vi "Programing Falsh.vi"() -> ()   [LabVIEW 2018]
uses:
  Typedefs/Command.ctl
  Sub'VIs/Typedefs/CaseControl.ctl
  <vilib>/xnet/xnet.llb/XNET Frame CAN.ctl
  <vilib>/xnet/xnet.llb/XNET Frame Type CAN.ctl
panel:
  in  "exit":bool
  out "Ops":string
  in  "CAN Interface":refnum<k21>="CAN1"
  in  "Start":bool
  in  "path":path
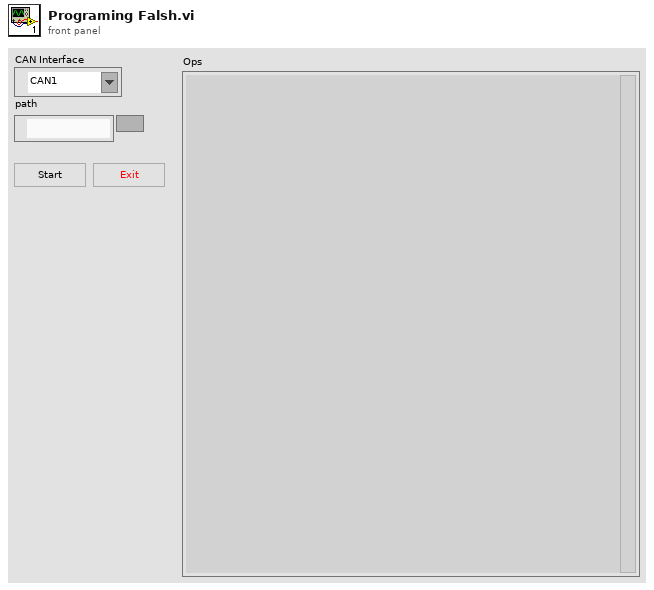
[diagram p1: front panel]
types:
  T1 = typedef "Command.ctl" = enum16{"Extend Session: 10 83", "Tester Present: 3E 80", "Resquest Seed: 27 01", "Send Key: 27 02", "Check FBL:  31 01 FD 02", "Control DTC: 85 82", "Comm Control: 28 83 01", "Program Session Request: 10 02", "Request Seed: 27 35", "Seed Key: 27 36", "Request Download: 34 00 44", "Transfer Data: 36 XX YY", "More Data?", "Request Transfer Exit: 37", "Check Flash Driver Validity: 01 FD 03", "More Segment?", "Write Data Fingereint: 23 F1 F0+26", "EraseFlashMemory Routine: 31 01 FD 00 44", "More segment?(each file)", "CheckAppSwAppData Validity: 31 01 FD 04 44", "CheckAppSwAppData Dependency: 31 01 fd 01", "ECU Reset: 11 81", "System: Init", "System: Idle", "System: Error", "System: Wait", "System: Delay", "System: CAN Send", "System: Exit"}
  T2 = typedef "CaseControl.ctl" = cluster{"histCase":cluster{"time":string, "event":T1, "pass?":bool}[], "retryCount":i32, "lastCase":T1, "nextEvent":T1}
  T3 = cluster{"Write Session in":refnum<k21>, "Read Session in":refnum<k21>, "TxRx Data":string[][], "Response Good?":bool, "spreadsheet string":string, "Rx Message":u8[]}
  T4 = cluster{"path":path, "CAN":cluster{"Write Session in":refnum<k21>, "Read Session in":refnum<k21>, "TxRx Data":string[][], "Response Good?":bool, "spreadsheet string":string, "Rx Message":u8[]}, "error":errorcluster, "CaseControl":T2, "Delay_ms":i32, "Nextevent":T1}
  T5 = typedef "XNET Frame CAN.ctl" = cluster{"timestamp":timestamp, "payload":u8[], "identifier":u32, "type":T6, "extended?":bool, "echo?":bool}
  T6 = typedef "XNET Frame Type CAN.ctl" = u8
  T7 = cluster{"time":string, "event":T1, "pass?":bool}[]
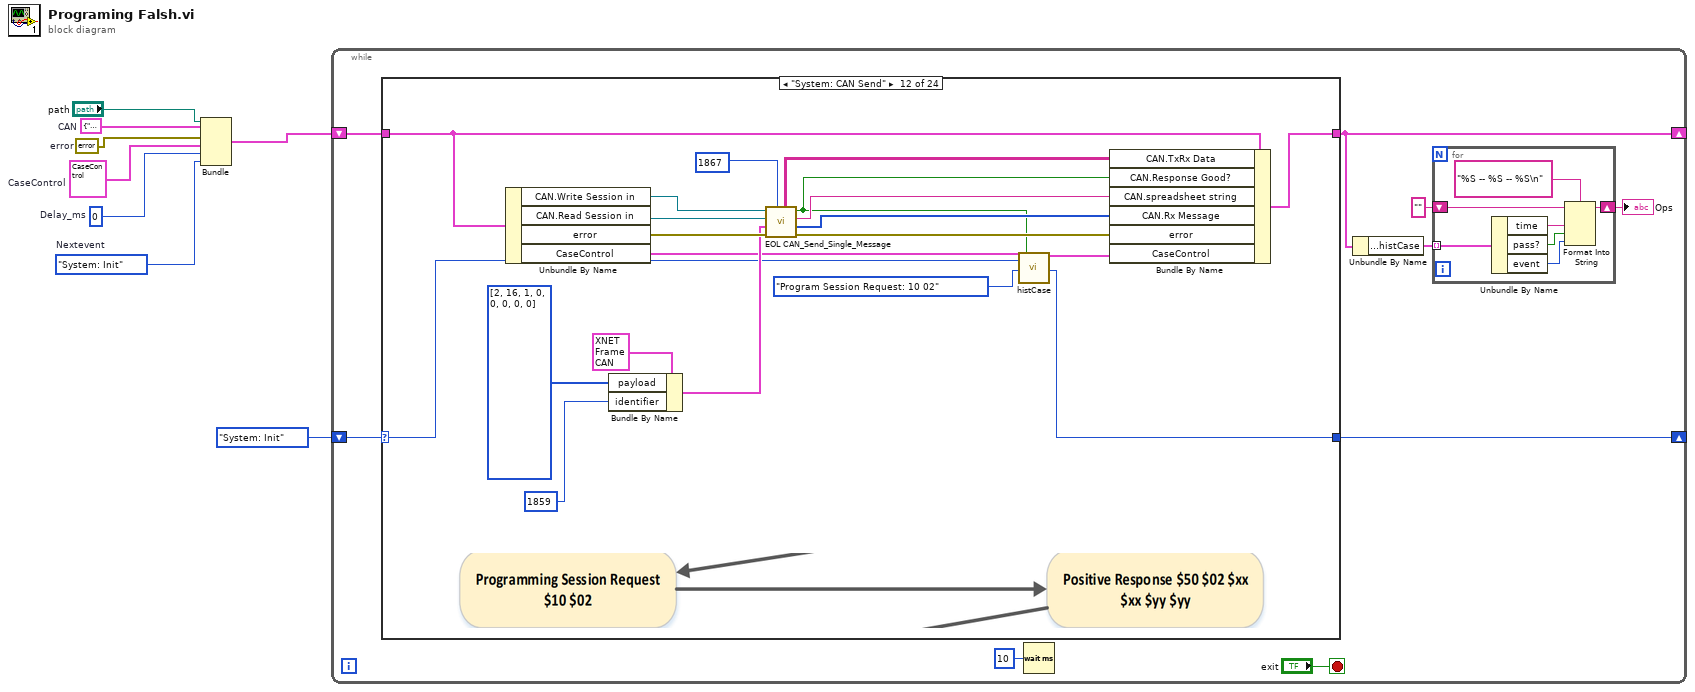
[diagram p0: block diagram]
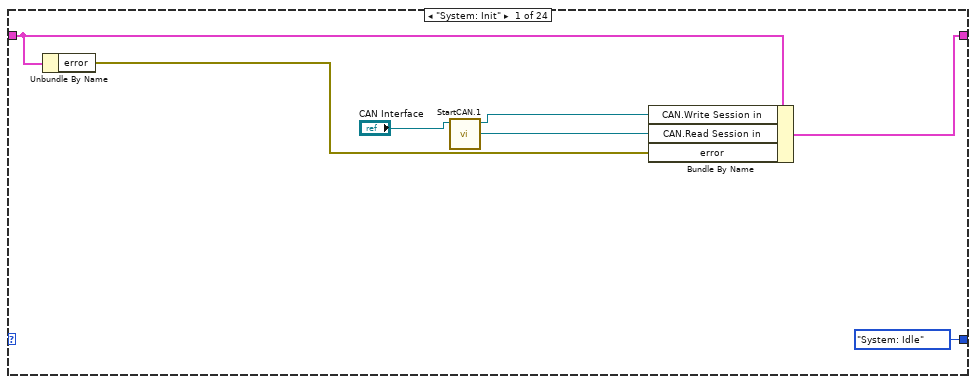
[diagram p2: hidden frame]
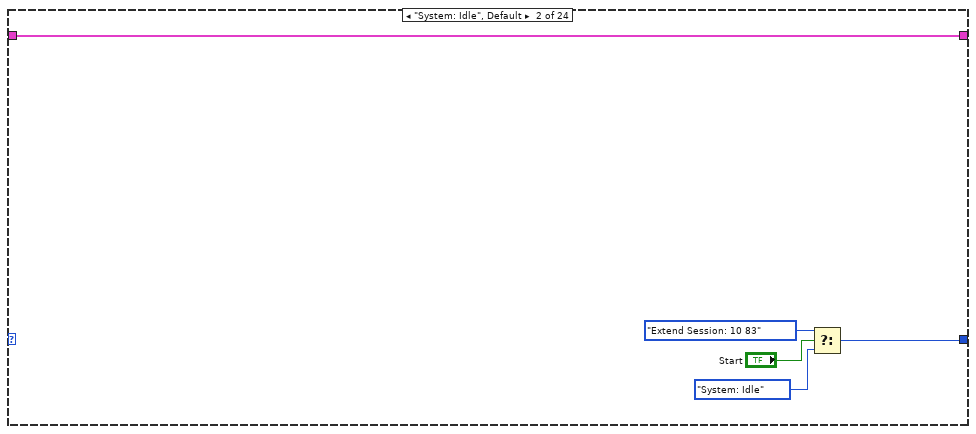
[diagram p3: hidden frame]
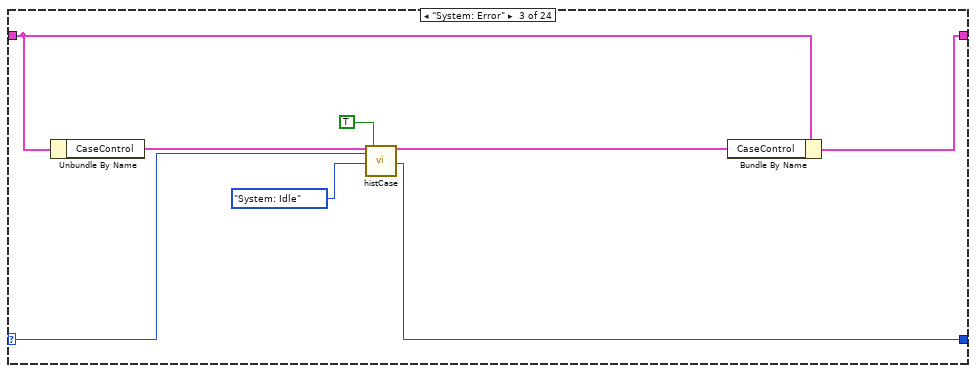
[diagram p4: hidden frame]
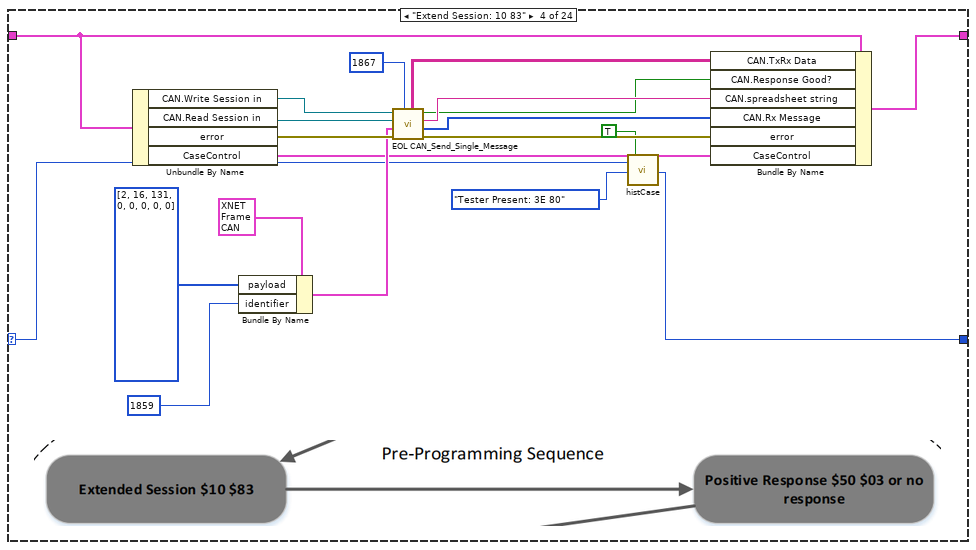
[diagram p5: hidden frame]
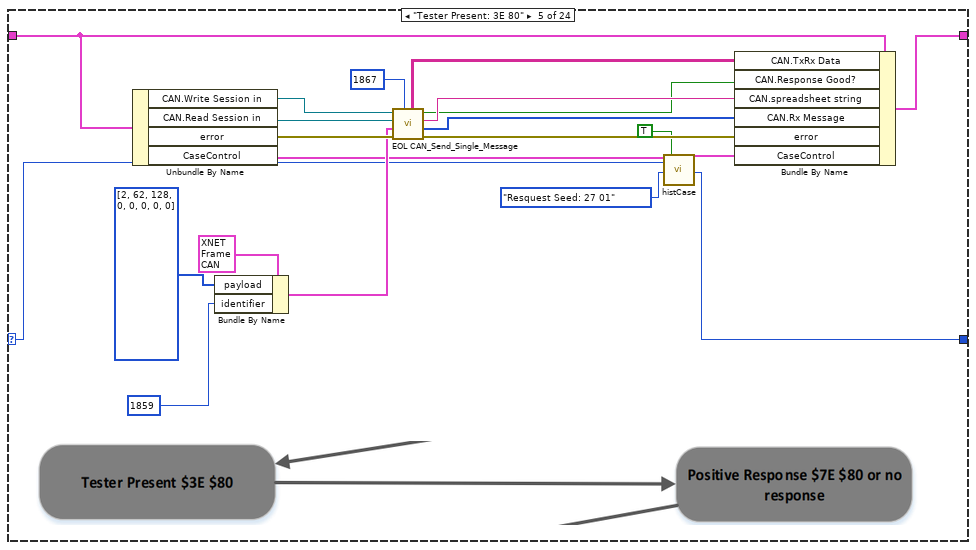
[diagram p6: hidden frame]
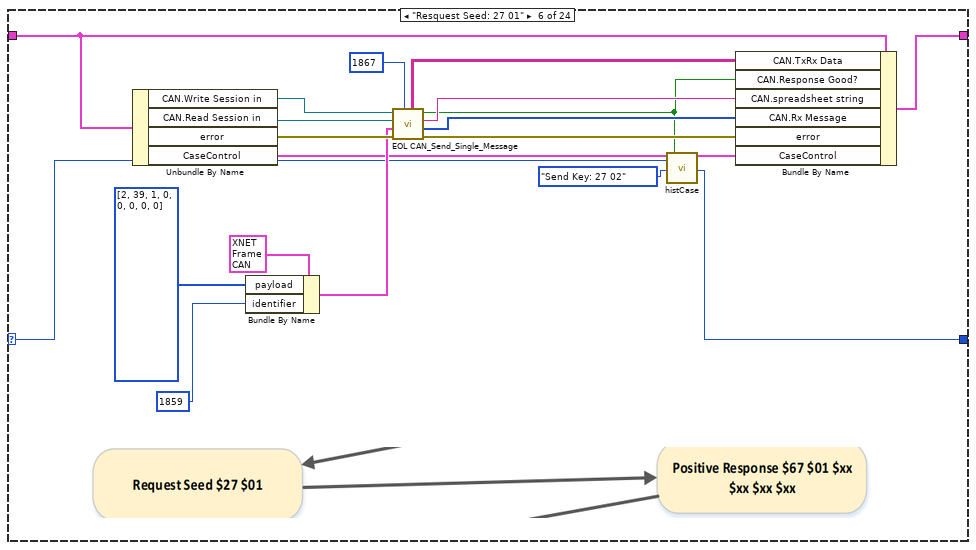
[diagram p7: hidden frame]
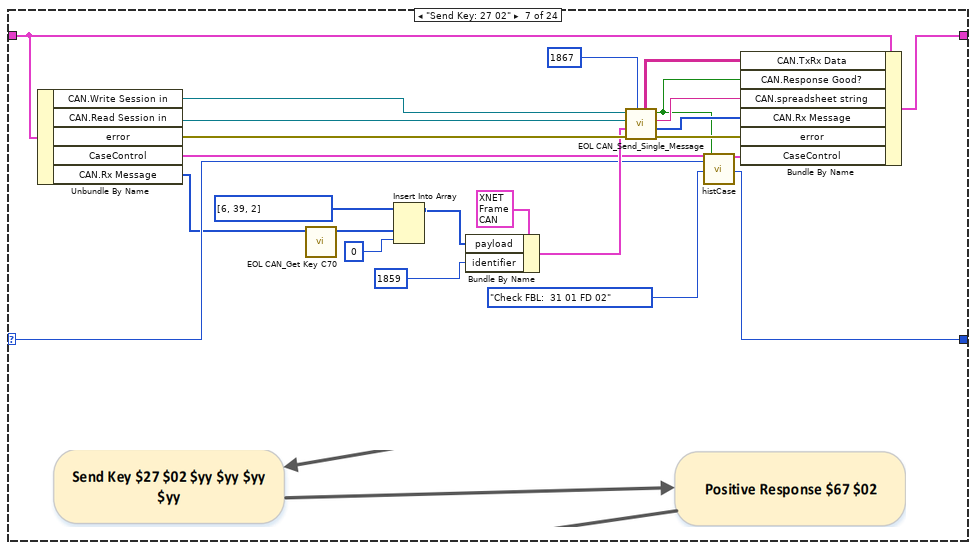
[diagram p8: hidden frame]
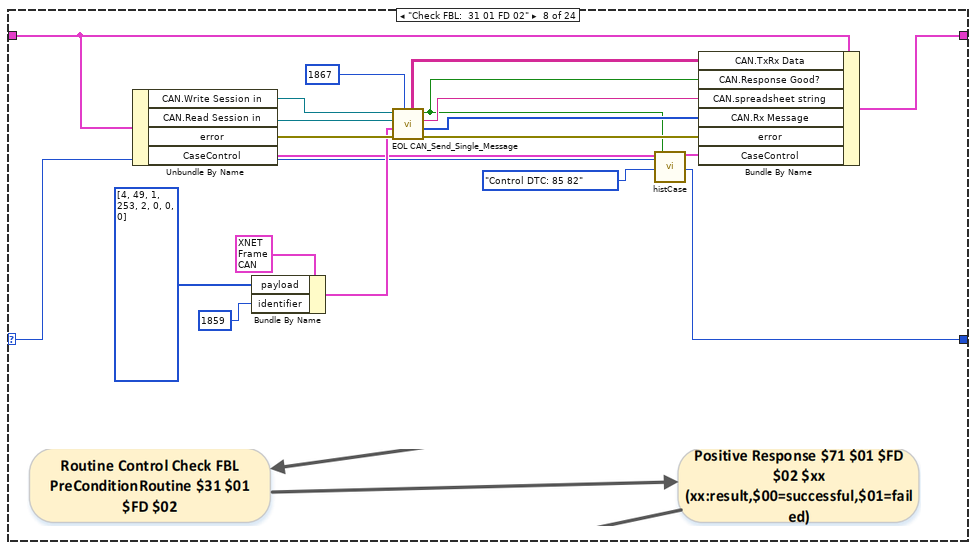
[diagram p9: hidden frame]
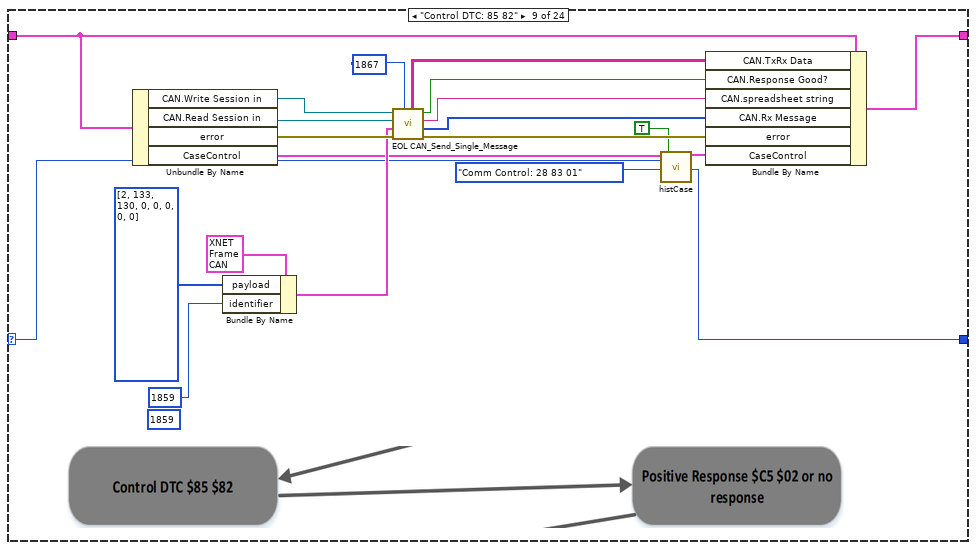
[diagram p10: hidden frame]
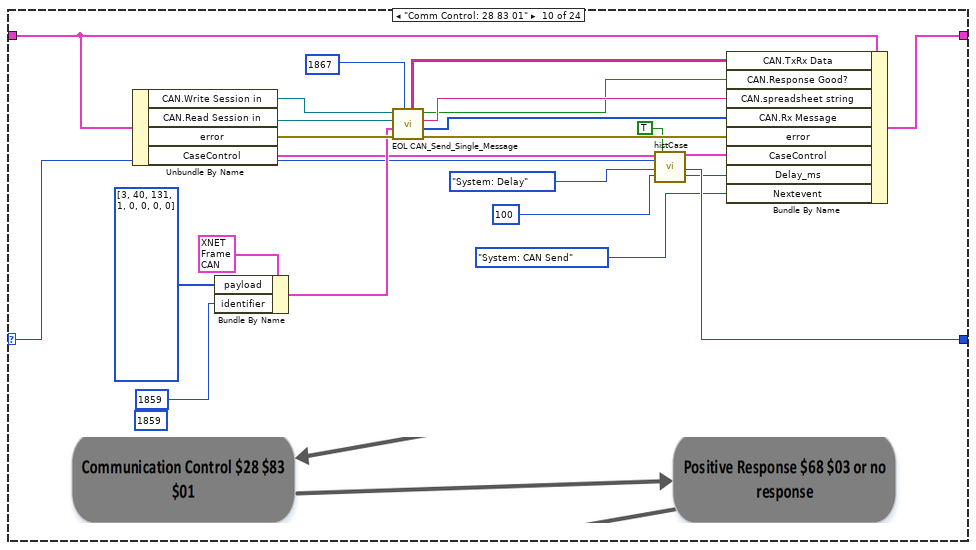
[diagram p11: hidden frame]
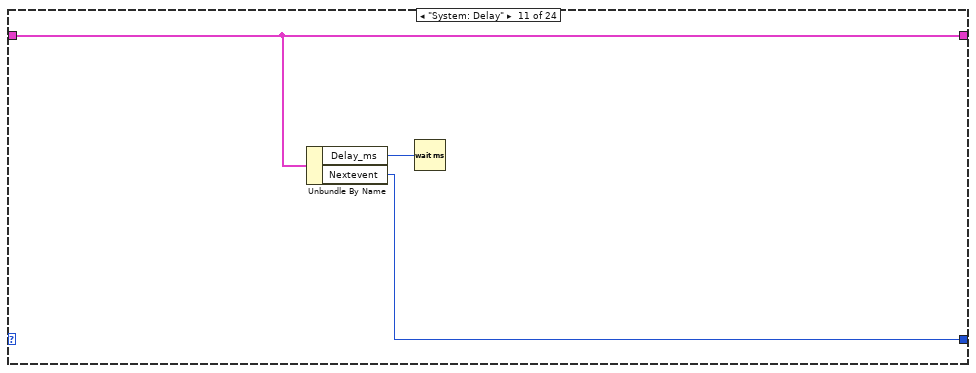
[diagram p12: hidden frame]
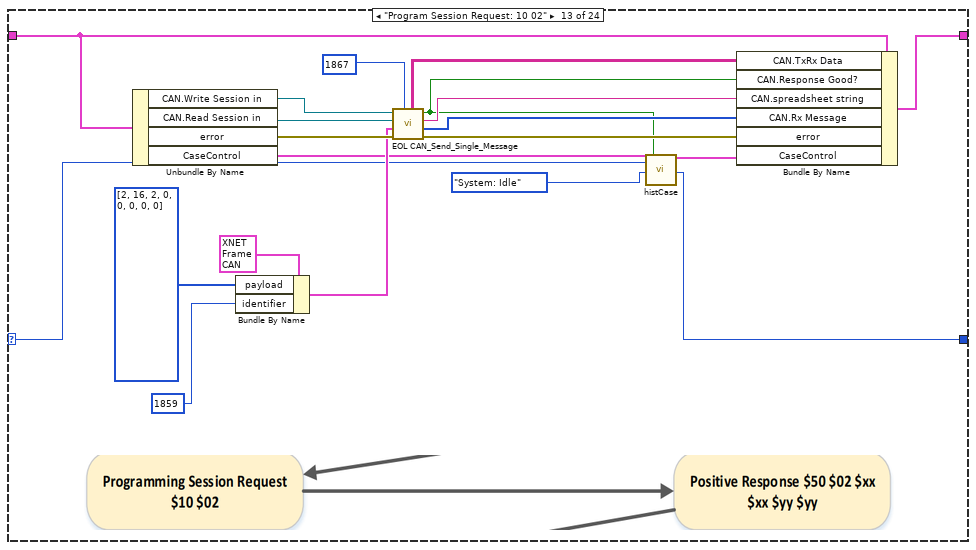
[diagram p13: hidden frame]
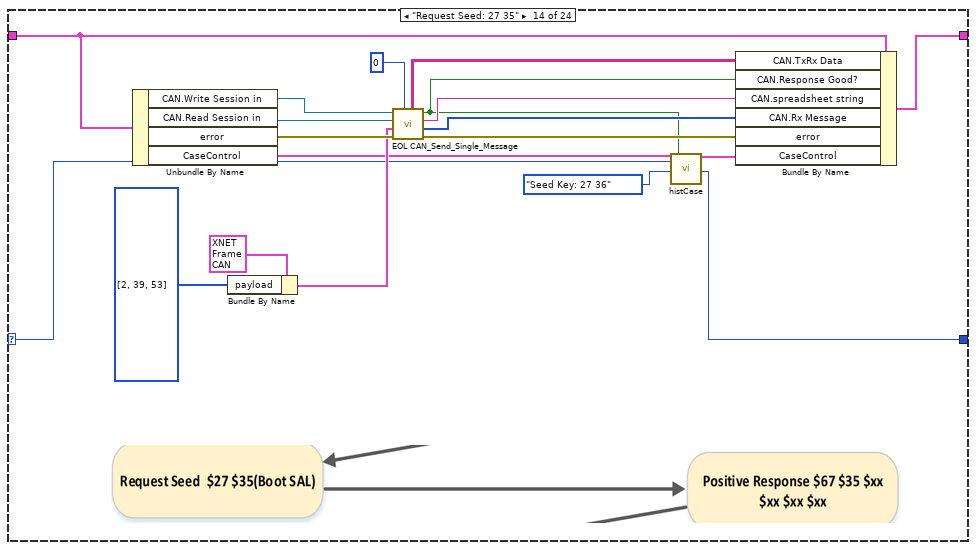
[diagram p14: hidden frame]
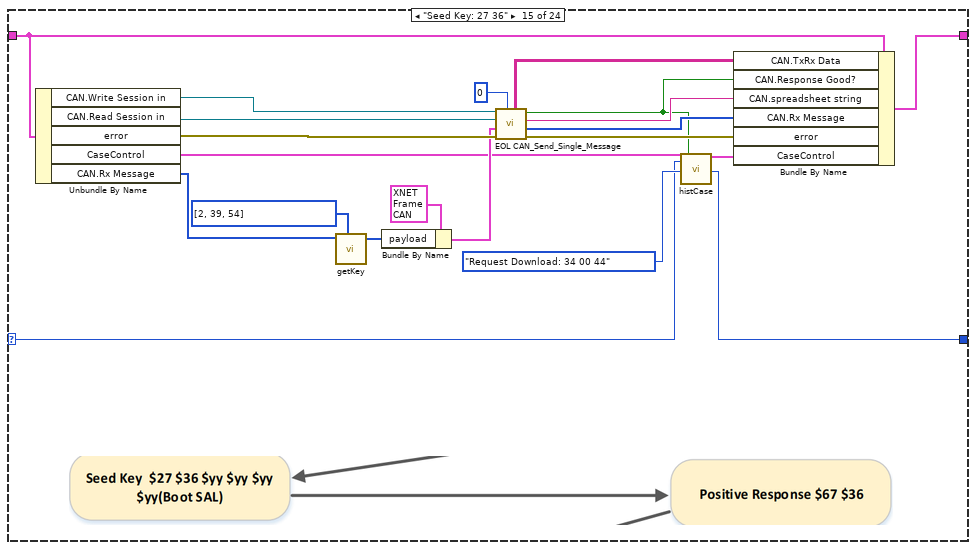
[diagram p15: hidden frame]
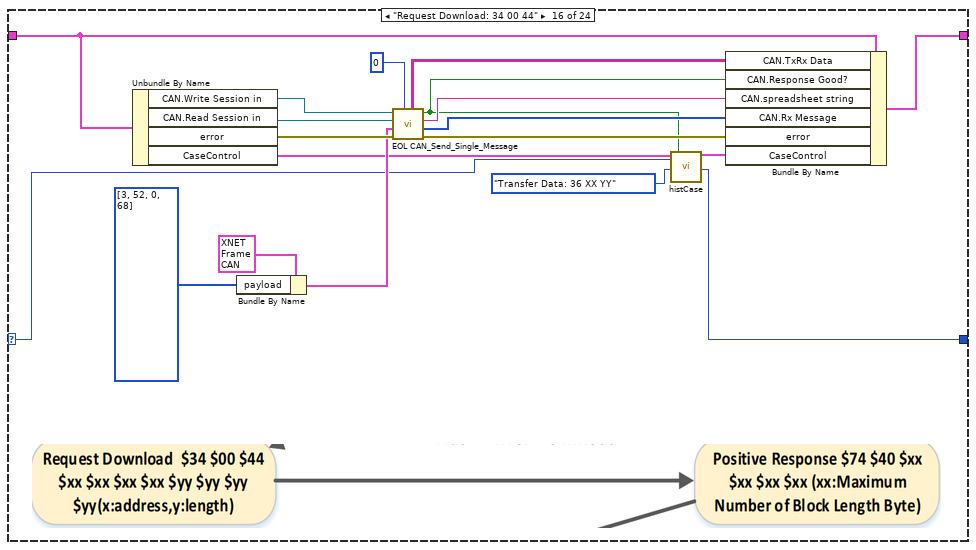
[diagram p16: hidden frame]
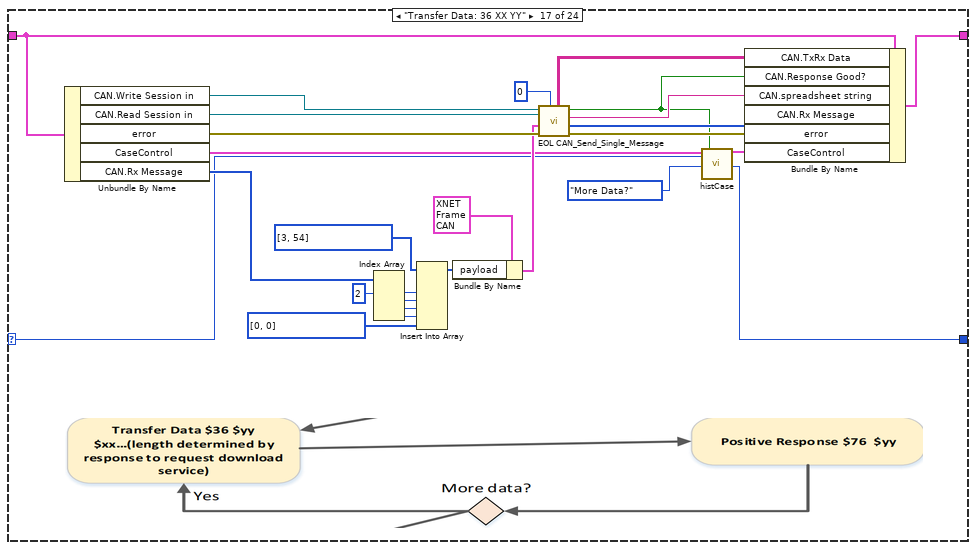
[diagram p17: hidden frame]
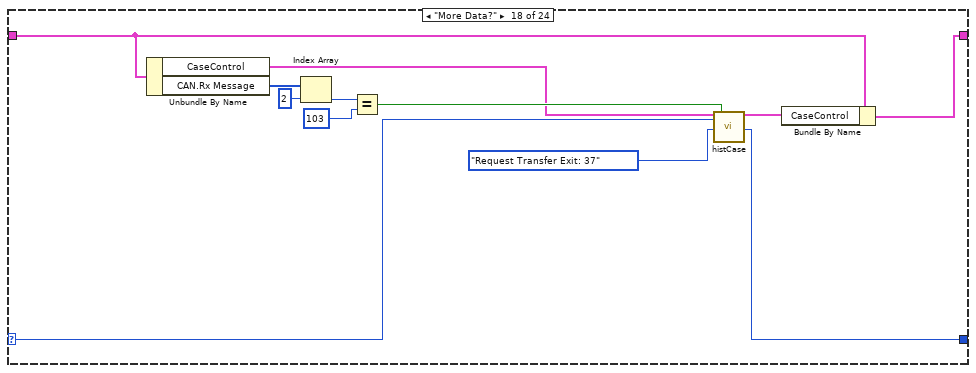
[diagram p18: hidden frame]
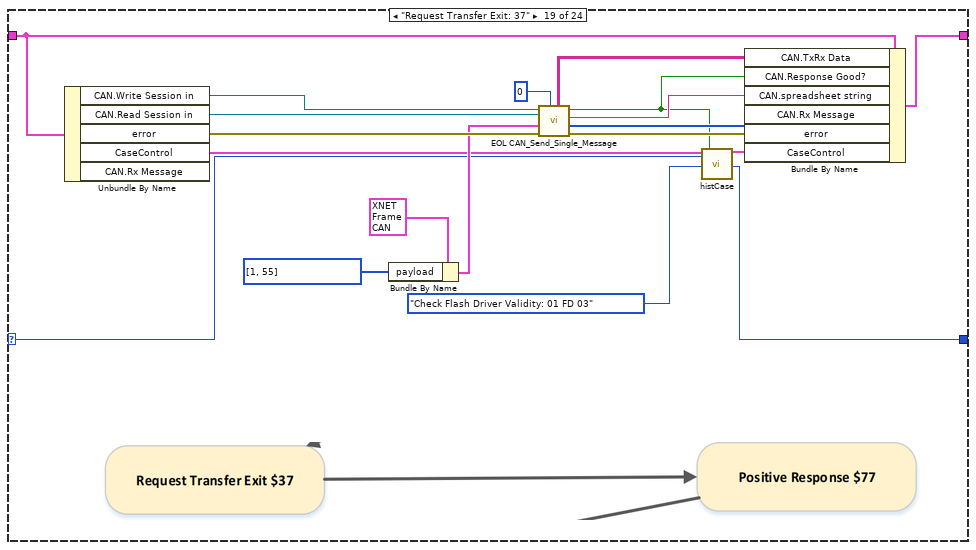
[diagram p19: hidden frame]
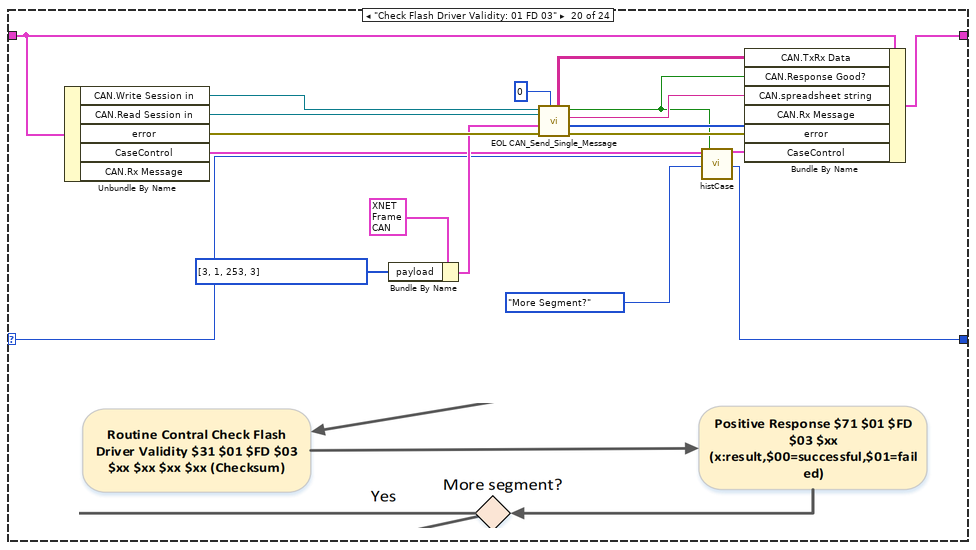
[diagram p20: hidden frame]
diagram:
  w1 = Command."System: Init"  # Nextevent
  w2 = 0  # Delay_ms
  w3 = T2 {"histCase"=[], "retryCount"=0, "lastCase"=enum."Extend Session: 10 83", "nextEvent"=enum."Extend Session: 10 83"}  # CaseControl
  w5 = errorcluster {"status"=FALSE, "code"=0, "source"=""}  # error
  w7 = T3 {"Write Session in"="", "Read Session in"="", "TxRx Data"=[], "Response Good?"=FALSE, "spreadsheet string"="", "Rx Message"=[]}  # CAN
  n1 = Bundle("path"="path", "CAN"=w7, "error"=w5, "CaseControl"=w3, "Delay_ms"=w2, "Nextevent"=w1) -> (w6:T4)  [unwired: 1 in]
  n2 = while {
    shift-right: [w11] -> _
    shift-left: w6 -> [w16]
    shift-right: [w15] -> _
    shift-left: Command."System: Init" -> [w17]
    stop <- "exit" stop-if-true
    n3 = case shown="\"System: CAN Send\"" w17 {
      selector: w17 -> [_ _ w42 w48 w69 w88 w114 w133 w154 w177 _ w200 w220 w238 w257 w278 w297 w324 w337 w356 w379 w390 w409 w432]
      tunnel: w16 -> [w31 w32 w41 w62 w83 w103 w127 w147 w168 w191 w197 w214 w234 w253 w274 w293 w320 w331 w351 w370 w384 w404 w423 w437]
      tunnel: [w30 w32 w39 w61 w82 w102 w126 w146 w167 w190 w197 w213 w233 w252 w273 w292 w319 w330 w350 w369 w383 w403 w422 w436] -> w11
      tunnel: [Command."System: Idle" ("event") w36 w38 w50 w71 w90 w117 w135 w156 w179 w195 w203 w223 w241 w259 w281 w300 w325 w340 w359 w380 w393 w412 w433] -> w15
      frame "System: Init" {
        n4 = Unbundle By Name(w31) -> ("error"=w28:errorcluster)
        n5 = call "StartCAN.1.vi"("CAN Interface"="CAN Interface") -> ("Read Session out"=w25:refnum<k21>, "DSC Write Session out"=w26:refnum<k21>)  [unwired: 7 in, 2 out]
        n6 = Bundle By Name(cluster=w31, "CAN.Write Session in"=w26, "CAN.Read Session in"=w25, "error"=w28) -> (w30:T4)
      }
      frame "System: Idle", Default {
        n7 = Select(t=Command."Extend Session: 10 83", s="Start", f=Command."System: Idle") -> (s? t:f=w36:T1)
      }
      frame "System: Error" {
        n8 = Unbundle By Name(w41) -> ("CaseControl"=w44:T2)
        n9 = call "histCase.vi"("CaseControl"=w44, "last case"=w42, "event"=Command."System: Idle", "finish?"=TRUE) -> ("CaseControl"=w40:T2, "event"=w38:T1)  [unwired: 14 in]
        n10 = Bundle By Name(cluster=w41, "CaseControl"=w40) -> (w39:T4)
      }
      frame "Extend Session: 10 83" {
        n11 = Unbundle By Name(w62) -> ("CAN.Write Session in"=w65:refnum<k21>, "CAN.Read Session in"=w64:refnum<k21>, "error"=w63:errorcluster, "CaseControl"=w52:T2)
        n12 = Bundle By Name(cluster=T5 {"timestamp"=timestamp(0 s since 1904-01-01), "payload"=[2, 39, 3, 85, 85, 85, 85, 85], "identifier"=402391172, "type"=0, "extended?"=FALSE, "echo?"=FALSE} ("Tx CAN frame"), "payload"=u8[] [2, 16, 131, 0, 0, 0, 0, 0], "identifier"=u32 1859) -> (w54:T5)
        n13 = call "EOL CAN_Send_Single_Message.vi"("Rx Arbitration Id"=u32 1867, "Error in"=w63, "Tx CAN frame"=w54, "Read Session in"=w64, "Write Session in"=w65) -> ("Error out"=w58:errorcluster, "Rx Message"=w59:u8[], "spreadsheet string"=w60:string, "Response Good?"=w46:bool, "TxRx Data"=w56:string[][])  [unwired: 2 in]
        n14 = call "histCase.vi"("CaseControl"=w52, "last case"=w48, "event"=Command."Tester Present: 3E 80", "finish?"=TRUE) -> ("CaseControl"=w51:T2, "event"=w50:T1)  [unwired: 14 in]
        n15 = Bundle By Name(cluster=w62, "CAN.TxRx Data"=w56, "CAN.Response Good?"=w46, "CAN.spreadsheet string"=w60, "CAN.Rx Message"=w59, "error"=w58, "CaseControl"=w51) -> (w61:T4)
      }
      frame "Tester Present: 3E 80" {
        n16 = Unbundle By Name(w83) -> ("CAN.Write Session in"=w86:refnum<k21>, "CAN.Read Session in"=w85:refnum<k21>, "error"=w84:errorcluster, "CaseControl"=w73:T2)
        n17 = Bundle By Name(cluster=T5 {"timestamp"=timestamp(0 s since 1904-01-01), "payload"=[2, 39, 3, 85, 85, 85, 85, 85], "identifier"=402391172, "type"=0, "extended?"=TRUE, "echo?"=FALSE} ("Tx CAN frame"), "payload"=u8[] [2, 62, 128, 0, 0, 0, 0, 0], "identifier"=u32 1859) -> (w76:T5)
        n18 = call "EOL CAN_Send_Single_Message.vi"("Rx Arbitration Id"=u32 1867, "Error in"=w84, "Tx CAN frame"=w76, "Read Session in"=w85, "Write Session in"=w86) -> ("Error out"=w79:errorcluster, "Rx Message"=w80:u8[], "spreadsheet string"=w81:string, "Response Good?"=w72:bool, "TxRx Data"=w78:string[][])  [unwired: 2 in]
        n19 = call "histCase.vi"("CaseControl"=w73, "last case"=w69, "event"=Command."Resquest Seed: 27 01", "finish?"=TRUE) -> ("CaseControl"=w74:T2, "event"=w71:T1)  [unwired: 14 in]
        n20 = Bundle By Name(cluster=w83, "CAN.TxRx Data"=w78, "CAN.Response Good?"=w72, "CAN.spreadsheet string"=w81, "CAN.Rx Message"=w80, "error"=w79, "CaseControl"=w74) -> (w82:T4)
      }
      frame "Resquest Seed: 27 01" {
        n21 = Unbundle By Name(w103) -> ("CAN.Write Session in"=w106:refnum<k21>, "CAN.Read Session in"=w105:refnum<k21>, "error"=w104:errorcluster, "CaseControl"=w93:T2)
        n22 = Bundle By Name(cluster=T5 {"timestamp"=timestamp(0 s since 1904-01-01), "payload"=[2, 39, 3, 85, 85, 85, 85, 85], "identifier"=402391172, "type"=0, "extended?"=TRUE, "echo?"=FALSE} ("Tx CAN frame"), "payload"=u8[] [2, 39, 1, 0, 0, 0, 0, 0], "identifier"=u32 1859) -> (w95:T5)
        n23 = call "EOL CAN_Send_Single_Message.vi"("Rx Arbitration Id"=u32 1867, "Error in"=w104, "Tx CAN frame"=w95, "Read Session in"=w105, "Write Session in"=w106) -> ("Error out"=w99:errorcluster, "Rx Message"=w100:u8[], "spreadsheet string"=w101:string, "Response Good?"=w91:bool, "TxRx Data"=w97:string[][])  [unwired: 2 in]
        n24 = call "histCase.vi"("CaseControl"=w93, "last case"=w88, "event"=Command."Send Key: 27 02", "finish?"=w91) -> ("CaseControl"=w92:T2, "event"=w90:T1)  [unwired: 14 in]
        n25 = Bundle By Name(cluster=w103, "CAN.TxRx Data"=w97, "CAN.Response Good?"=w91, "CAN.spreadsheet string"=w101, "CAN.Rx Message"=w100, "error"=w99, "CaseControl"=w92) -> (w102:T4)
      }
      frame "Send Key: 27 02" {
        n26 = Unbundle By Name(w127) -> ("CAN.Write Session in"=w130:refnum<k21>, "CAN.Read Session in"=w129:refnum<k21>, "error"=w128:errorcluster, "CaseControl"=w119:T2, "CAN.Rx Message"=w112:u8[])
        n27 = call "EOL CAN_Get Key C70.vi"("Seed message"=w112) -> ("Key"=w109:u32[])  [unwired: 10 in]
        n28 = Insert Into Array(array=u8[] [6, 39, 2] ("payload"), new element #1=w109, new element #2=u8 0 ("新元素/子数组")) -> (w107:u8[])  [unwired: 1 in]
        n29 = Bundle By Name(cluster=T5 {"timestamp"=timestamp(0 s since 1904-01-01), "payload"=[2, 39, 3, 85, 85, 85, 85, 85], "identifier"=402391172, "type"=0, "extended?"=TRUE, "echo?"=FALSE} ("Tx CAN frame"), "payload"=w107, "identifier"=u32 1859) -> (w120:T5)
        n30 = call "EOL CAN_Send_Single_Message.vi"("Rx Arbitration Id"=u32 1867, "Error in"=w128, "Tx CAN frame"=w120, "Read Session in"=w129, "Write Session in"=w130) -> ("Error out"=w123:errorcluster, "Rx Message"=w124:u8[], "spreadsheet string"=w125:string, "Response Good?"=w115:bool, "TxRx Data"=w122:string[][])  [unwired: 2 in]
        n31 = call "histCase.vi"("CaseControl"=w119, "last case"=w114, "event"=Command."Check FBL:  31 01 FD 02", "finish?"=w115) -> ("CaseControl"=w118:T2, "event"=w117:T1)  [unwired: 14 in]
        n32 = Bundle By Name(cluster=w127, "CAN.TxRx Data"=w122, "CAN.Response Good?"=w115, "CAN.spreadsheet string"=w125, "CAN.Rx Message"=w124, "error"=w123, "CaseControl"=w118) -> (w126:T4)
      }
      frame "Check FBL:  31 01 FD 02" {
        n33 = Unbundle By Name(w147) -> ("CAN.Write Session in"=w150:refnum<k21>, "CAN.Read Session in"=w149:refnum<k21>, "error"=w148:errorcluster, "CaseControl"=w138:T2)
        n34 = Bundle By Name(cluster=T5 {"timestamp"=timestamp(0 s since 1904-01-01), "payload"=[2, 39, 3, 85, 85, 85, 85, 85], "identifier"=402391172, "type"=0, "extended?"=TRUE, "echo?"=FALSE} ("Tx CAN frame"), "payload"=u8[] [4, 49, 1, 253, 2, 0, 0, 0], "identifier"=u32 1859) -> (w140:T5)
        n35 = call "EOL CAN_Send_Single_Message.vi"("Rx Arbitration Id"=u32 1867, "Error in"=w148, "Tx CAN frame"=w140, "Read Session in"=w149, "Write Session in"=w150) -> ("Error out"=w143:errorcluster, "Rx Message"=w144:u8[], "spreadsheet string"=w145:string, "Response Good?"=w136:bool, "TxRx Data"=w142:string[][])  [unwired: 2 in]
        n36 = call "histCase.vi"("CaseControl"=w138, "last case"=w133, "event"=Command."Control DTC: 85 82", "finish?"=w136) -> ("CaseControl"=w137:T2, "event"=w135:T1)  [unwired: 14 in]
        n37 = Bundle By Name(cluster=w147, "CAN.TxRx Data"=w142, "CAN.Response Good?"=w136, "CAN.spreadsheet string"=w145, "CAN.Rx Message"=w144, "error"=w143, "CaseControl"=w137) -> (w146:T4)
      }
      frame "Control DTC: 85 82" {
        (unwired) u32 1859 ("identifier")
        n38 = Unbundle By Name(w168) -> ("CAN.Write Session in"=w171:refnum<k21>, "CAN.Read Session in"=w170:refnum<k21>, "error"=w169:errorcluster, "CaseControl"=w159:T2)
        n39 = Bundle By Name(cluster=T5 {"timestamp"=timestamp(0 s since 1904-01-01), "payload"=[2, 39, 3, 85, 85, 85, 85, 85], "identifier"=402391172, "type"=0, "extended?"=TRUE, "echo?"=FALSE} ("Tx CAN frame"), "payload"=u8[] [2, 133, 130, 0, 0, 0, 0, 0], "identifier"=u32 1859) -> (w161:T5)
        n40 = call "EOL CAN_Send_Single_Message.vi"("Rx Arbitration Id"=u32 1867, "Error in"=w169, "Tx CAN frame"=w161, "Read Session in"=w170, "Write Session in"=w171) -> ("Error out"=w164:errorcluster, "Rx Message"=w165:u8[], "spreadsheet string"=w166:string, "Response Good?"=w157:bool, "TxRx Data"=w163:string[][])  [unwired: 2 in]
        n41 = call "histCase.vi"("CaseControl"=w159, "last case"=w154, "event"=Command."Comm Control: 28 83 01", "finish?"=TRUE) -> ("CaseControl"=w158:T2, "event"=w156:T1)  [unwired: 14 in]
        n42 = Bundle By Name(cluster=w168, "CAN.TxRx Data"=w163, "CAN.Response Good?"=w157, "CAN.spreadsheet string"=w166, "CAN.Rx Message"=w165, "error"=w164, "CaseControl"=w158) -> (w167:T4)
      }
      frame "Comm Control: 28 83 01" {
        (unwired) u32 1859 ("identifier")
        n43 = Unbundle By Name(w191) -> ("CAN.Write Session in"=w194:refnum<k21>, "CAN.Read Session in"=w193:refnum<k21>, "error"=w192:errorcluster, "CaseControl"=w182:T2)
        n44 = Bundle By Name(cluster=T5 {"timestamp"=timestamp(0 s since 1904-01-01), "payload"=[2, 39, 3, 85, 85, 85, 85, 85], "identifier"=402391172, "type"=0, "extended?"=TRUE, "echo?"=FALSE} ("Tx CAN frame"), "payload"=u8[] [3, 40, 131, 1, 0, 0, 0, 0], "identifier"=u32 1859) -> (w184:T5)
        n45 = call "EOL CAN_Send_Single_Message.vi"("Rx Arbitration Id"=u32 1867, "Error in"=w192, "Tx CAN frame"=w184, "Read Session in"=w193, "Write Session in"=w194) -> ("Error out"=w187:errorcluster, "Rx Message"=w188:u8[], "spreadsheet string"=w189:string, "Response Good?"=w180:bool, "TxRx Data"=w186:string[][])  [unwired: 2 in]
        n46 = call "histCase.vi"("CaseControl"=w182, "last case"=w177, "event"=Command."System: Delay", "finish?"=TRUE) -> ("CaseControl"=w181:T2, "event"=w179:T1)  [unwired: 14 in]
        n47 = Bundle By Name(cluster=w191, "CAN.TxRx Data"=w186, "CAN.Response Good?"=w180, "CAN.spreadsheet string"=w189, "CAN.Rx Message"=w188, "error"=w187, "CaseControl"=w181, "Delay_ms"=100, "Nextevent"=Command."System: CAN Send") -> (w190:T4)
      }
      frame "System: Delay" {
        n48 = Unbundle By Name(w197) -> ("Delay_ms"=w196:i32, "Nextevent"=w195:T1)
        n49 = Wait (ms)(milliseconds to wait=w196) -> ()  [unwired: 1 out]
      }
      frame "System: CAN Send" {
        n50 = Unbundle By Name(w214) -> ("CAN.Write Session in"=w217:refnum<k21>, "CAN.Read Session in"=w216:refnum<k21>, "error"=w215:errorcluster, "CaseControl"=w205:T2)
        n51 = Bundle By Name(cluster=T5 {"timestamp"=timestamp(0 s since 1904-01-01), "payload"=[2, 39, 3, 85, 85, 85, 85, 85], "identifier"=402391172, "type"=0, "extended?"=TRUE, "echo?"=FALSE} ("Tx CAN frame"), "payload"=u8[] [2, 16, 1, 0, 0, 0, 0, 0], "identifier"=u32 1859) -> (w207:T5)
        n52 = call "EOL CAN_Send_Single_Message.vi"("Rx Arbitration Id"=u32 1867, "Error in"=w215, "Tx CAN frame"=w207, "Read Session in"=w216, "Write Session in"=w217) -> ("Error out"=w210:errorcluster, "Rx Message"=w211:u8[], "spreadsheet string"=w212:string, "Response Good?"=w201:bool, "TxRx Data"=w209:string[][])  [unwired: 2 in]
        n53 = call "histCase.vi"("CaseControl"=w205, "last case"=w200, "event"=Command."Program Session Request: 10 02", "finish?"=w201) -> ("CaseControl"=w204:T2, "event"=w203:T1)  [unwired: 14 in]
        n54 = Bundle By Name(cluster=w214, "CAN.TxRx Data"=w209, "CAN.Response Good?"=w201, "CAN.spreadsheet string"=w212, "CAN.Rx Message"=w211, "error"=w210, "CaseControl"=w204) -> (w213:T4)
      }
      frame "Program Session Request: 10 02" {
        n55 = Unbundle By Name(w234) -> ("CAN.Write Session in"=w237:refnum<k21>, "CAN.Read Session in"=w236:refnum<k21>, "error"=w235:errorcluster, "CaseControl"=w225:T2)
        n56 = Bundle By Name(cluster=T5 {"timestamp"=timestamp(0 s since 1904-01-01), "payload"=[2, 39, 3, 85, 85, 85, 85, 85], "identifier"=402391172, "type"=0, "extended?"=TRUE, "echo?"=FALSE} ("Tx CAN frame"), "payload"=u8[] [2, 16, 2, 0, 0, 0, 0, 0], "identifier"=u32 1859) -> (w227:T5)
        n57 = call "EOL CAN_Send_Single_Message.vi"("Rx Arbitration Id"=u32 1867, "Error in"=w235, "Tx CAN frame"=w227, "Read Session in"=w236, "Write Session in"=w237) -> ("Error out"=w230:errorcluster, "Rx Message"=w231:u8[], "spreadsheet string"=w232:string, "Response Good?"=w221:bool, "TxRx Data"=w229:string[][])  [unwired: 2 in]
        n58 = call "histCase.vi"("CaseControl"=w225, "last case"=w220, "event"=Command."System: Idle", "finish?"=w221) -> ("CaseControl"=w224:T2, "event"=w223:T1)  [unwired: 14 in]
        n59 = Bundle By Name(cluster=w234, "CAN.TxRx Data"=w229, "CAN.Response Good?"=w221, "CAN.spreadsheet string"=w232, "CAN.Rx Message"=w231, "error"=w230, "CaseControl"=w224) -> (w233:T4)
      }
      frame "Request Seed: 27 35" {
        n60 = Unbundle By Name(w253) -> ("CAN.Write Session in"=w256:refnum<k21>, "CAN.Read Session in"=w255:refnum<k21>, "error"=w254:errorcluster, "CaseControl"=w243:T2)
        n61 = Bundle By Name(cluster=T5 {"timestamp"=timestamp(0 s since 1904-01-01), "payload"=[2, 39, 3, 85, 85, 85, 85, 85], "identifier"=402391172, "type"=0, "extended?"=TRUE, "echo?"=FALSE} ("Tx CAN frame"), "payload"=u8[] [2, 39, 53]) -> (w245:T5)
        n62 = call "EOL CAN_Send_Single_Message.vi"("Rx Arbitration Id"=u32 0, "Error in"=w254, "Tx CAN frame"=w245, "Read Session in"=w255, "Write Session in"=w256) -> ("Error out"=w249:errorcluster, "Rx Message"=w250:u8[], "spreadsheet string"=w251:string, "Response Good?"=w239:bool, "TxRx Data"=w247:string[][])  [unwired: 2 in]
        n63 = call "histCase.vi"("CaseControl"=w243, "last case"=w238, "event"=Command."Seed Key: 27 36", "finish?"=w239) -> ("CaseControl"=w242:T2, "event"=w241:T1)  [unwired: 14 in]
        n64 = Bundle By Name(cluster=w253, "CAN.TxRx Data"=w247, "CAN.Response Good?"=w239, "CAN.spreadsheet string"=w251, "CAN.Rx Message"=w250, "error"=w249, "CaseControl"=w242) -> (w252:T4)
      }
      frame "Seed Key: 27 36" {
        n65 = Unbundle By Name(w274) -> ("CAN.Write Session in"=w277:refnum<k21>, "CAN.Read Session in"=w276:refnum<k21>, "error"=w275:errorcluster, "CaseControl"=w262:T2, "CAN.Rx Message"=w263:u8[])
        n66 = call "getKey.vi"("payload"=u8[] [2, 39, 54], "Rx"=w263) -> ("Keyload"=w264:u8[])  [unwired: 9 in]
        n67 = Bundle By Name(cluster=T5 {"timestamp"=timestamp(0 s since 1904-01-01), "payload"=[2, 39, 3, 85, 85, 85, 85, 85], "identifier"=402391172, "type"=0, "extended?"=TRUE, "echo?"=FALSE} ("Tx CAN frame"), "payload"=w264) -> (w266:T5)
        n68 = call "EOL CAN_Send_Single_Message.vi"("Rx Arbitration Id"=u32 0, "Error in"=w275, "Tx CAN frame"=w266, "Read Session in"=w276, "Write Session in"=w277) -> ("Error out"=w270:errorcluster, "Rx Message"=w271:u8[], "spreadsheet string"=w272:string, "Response Good?"=w260:bool, "TxRx Data"=w268:string[][])  [unwired: 2 in]
        n69 = call "histCase.vi"("CaseControl"=w262, "last case"=w257, "event"=Command."Request Download: 34 00 44", "finish?"=w260) -> ("CaseControl"=w261:T2, "event"=w259:T1)  [unwired: 14 in]
        n70 = Bundle By Name(cluster=w274, "CAN.TxRx Data"=w268, "CAN.Response Good?"=w260, "CAN.spreadsheet string"=w272, "CAN.Rx Message"=w271, "error"=w270, "CaseControl"=w261) -> (w273:T4)
      }
      frame "Request Download: 34 00 44" {
        n71 = Unbundle By Name(w293) -> ("CAN.Write Session in"=w296:refnum<k21>, "CAN.Read Session in"=w295:refnum<k21>, "error"=w294:errorcluster, "CaseControl"=w283:T2)
        n72 = Bundle By Name(cluster=T5 {"timestamp"=timestamp(0 s since 1904-01-01), "payload"=[2, 39, 3, 85, 85, 85, 85, 85], "identifier"=402391172, "type"=0, "extended?"=TRUE, "echo?"=FALSE} ("Tx CAN frame"), "payload"=u8[] [3, 52, 0, 68]) -> (w285:T5)
        n73 = call "EOL CAN_Send_Single_Message.vi"("Rx Arbitration Id"=u32 0, "Error in"=w294, "Tx CAN frame"=w285, "Read Session in"=w295, "Write Session in"=w296) -> ("Error out"=w289:errorcluster, "Rx Message"=w290:u8[], "spreadsheet string"=w291:string, "Response Good?"=w280:bool, "TxRx Data"=w287:string[][])  [unwired: 2 in]
        n74 = call "histCase.vi"("CaseControl"=w283, "last case"=w278, "event"=Command."Transfer Data: 36 XX YY", "finish?"=w280) -> ("CaseControl"=w282:T2, "event"=w281:T1)  [unwired: 14 in]
        n75 = Bundle By Name(cluster=w293, "CAN.TxRx Data"=w287, "CAN.Response Good?"=w280, "CAN.spreadsheet string"=w291, "CAN.Rx Message"=w290, "error"=w289, "CaseControl"=w282) -> (w292:T4)
      }
      frame "Transfer Data: 36 XX YY" {
        n76 = Unbundle By Name(w320) -> ("CAN.Write Session in"=w323:refnum<k21>, "CAN.Read Session in"=w322:refnum<k21>, "error"=w321:errorcluster, "CaseControl"=w302:T2, "CAN.Rx Message"=w311:u8[])
        n77 = Index Array(array=w311, index #1=2 ("索引")) -> (element #1=w308:u8, element #2=w307:u8, element #3=w306:u8, element #4=w305:u8)  [unwired: 3 in]
        n78 = Insert Into Array(array=u8[] [3, 54] ("payload"), new element #1=w308, new element #2=w307, new element #3=w306, new element #4=w305, new element #5=u8[] [0, 0] ("payload")) -> (w304:u8[])  [unwired: 1 in]
        n79 = Bundle By Name(cluster=T5 {"timestamp"=timestamp(0 s since 1904-01-01), "payload"=[2, 39, 3, 85, 85, 85, 85, 85], "identifier"=402391172, "type"=0, "extended?"=TRUE, "echo?"=FALSE} ("Tx CAN frame"), "payload"=w304) -> (w312:T5)
        n80 = call "EOL CAN_Send_Single_Message.vi"("Rx Arbitration Id"=u32 0, "Error in"=w321, "Tx CAN frame"=w312, "Read Session in"=w322, "Write Session in"=w323) -> ("Error out"=w316:errorcluster, "Rx Message"=w317:u8[], "spreadsheet string"=w318:string, "Response Good?"=w298:bool, "TxRx Data"=w314:string[][])  [unwired: 2 in]
        n81 = call "histCase.vi"("CaseControl"=w302, "last case"=w297, "event"=Command."More Data?", "finish?"=w298) -> ("CaseControl"=w301:T2, "event"=w300:T1)  [unwired: 14 in]
        n82 = Bundle By Name(cluster=w320, "CAN.TxRx Data"=w314, "CAN.Response Good?"=w298, "CAN.spreadsheet string"=w318, "CAN.Rx Message"=w317, "error"=w316, "CaseControl"=w301) -> (w319:T4)
      }
      frame "More Data?" {
        n83 = Unbundle By Name(w331) -> ("CaseControl"=w326:T2, "CAN.Rx Message"=w335:u8[])
        n84 = Index Array(array=w335, index=2 ("索引")) -> (element=w333:u8)
        n85 = Equal?(x=w333, y=103) -> (x = y?=w328:bool)
        n86 = call "histCase.vi"("CaseControl"=w326, "last case"=w324, "event"=Command."Request Transfer Exit: 37", "finish?"=w328) -> ("CaseControl"=w329:T2, "event"=w325:T1)  [unwired: 14 in]
        n87 = Bundle By Name(cluster=w331, "CaseControl"=w329) -> (w330:T4)
      }
      frame "Request Transfer Exit: 37" {
        n88 = Unbundle By Name(w351) -> ("CAN.Write Session in"=w354:refnum<k21>, "CAN.Read Session in"=w353:refnum<k21>, "error"=w352:errorcluster, "CaseControl"=w342:T2)  [unwired: 1 out]
        n89 = Bundle By Name(cluster=T5 {"timestamp"=timestamp(0 s since 1904-01-01), "payload"=[2, 39, 3, 85, 85, 85, 85, 85], "identifier"=402391172, "type"=0, "extended?"=TRUE, "echo?"=FALSE} ("Tx CAN frame"), "payload"=u8[] [1, 55]) -> (w343:T5)
        n90 = call "EOL CAN_Send_Single_Message.vi"("Rx Arbitration Id"=u32 0, "Error in"=w352, "Tx CAN frame"=w343, "Read Session in"=w353, "Write Session in"=w354) -> ("Error out"=w347:errorcluster, "Rx Message"=w348:u8[], "spreadsheet string"=w349:string, "Response Good?"=w338:bool, "TxRx Data"=w345:string[][])  [unwired: 2 in]
        n91 = call "histCase.vi"("CaseControl"=w342, "last case"=w337, "event"=Command."Check Flash Driver Validity: 01 FD 03", "finish?"=w338) -> ("CaseControl"=w341:T2, "event"=w340:T1)  [unwired: 14 in]
        n92 = Bundle By Name(cluster=w351, "CAN.TxRx Data"=w345, "CAN.Response Good?"=w338, "CAN.spreadsheet string"=w349, "CAN.Rx Message"=w348, "error"=w347, "CaseControl"=w341) -> (w350:T4)
      }
      frame "Check Flash Driver Validity: 01 FD 03" {
        n93 = Unbundle By Name(w370) -> ("CAN.Write Session in"=w373:refnum<k21>, "CAN.Read Session in"=w372:refnum<k21>, "error"=w371:errorcluster, "CaseControl"=w361:T2)  [unwired: 1 out]
        n94 = Bundle By Name(cluster=T5 {"timestamp"=timestamp(0 s since 1904-01-01), "payload"=[2, 39, 3, 85, 85, 85, 85, 85], "identifier"=402391172, "type"=0, "extended?"=TRUE, "echo?"=FALSE} ("Tx CAN frame"), "payload"=u8[] [3, 1, 253, 3]) -> (w362:T5)
        n95 = call "EOL CAN_Send_Single_Message.vi"("Rx Arbitration Id"=u32 0, "Error in"=w371, "Tx CAN frame"=w362, "Read Session in"=w372, "Write Session in"=w373) -> ("Error out"=w366:errorcluster, "Rx Message"=w367:u8[], "spreadsheet string"=w368:string, "Response Good?"=w357:bool, "TxRx Data"=w364:string[][])  [unwired: 2 in]
        n96 = call "histCase.vi"("CaseControl"=w361, "last case"=w356, "event"=Command."More Segment?", "finish?"=w357) -> ("CaseControl"=w360:T2, "event"=w359:T1)  [unwired: 14 in]
        n97 = Bundle By Name(cluster=w370, "CAN.TxRx Data"=w364, "CAN.Response Good?"=w357, "CAN.spreadsheet string"=w368, "CAN.Rx Message"=w367, "error"=w366, "CaseControl"=w360) -> (w369:T4)
      }
      frame "More Segment?" {
        n98 = Unbundle By Name(w384) -> ("CaseControl"=w381:T2, "CAN.Rx Message"=w388:u8[])
        n99 = Index Array(array=w388, index=5 ("索引")) -> (element=w386:u8)
        n100 = Equal?(x=w386, y=0) -> (x = y?=w378:bool)
        n101 = Select(t=Command."Write Data Fingereint: 23 F1 F0+26", s=w378, f=Command."Request Download: 34 00 44") -> (s? t:f=w375:T1)
        n102 = call "histCase.vi"("CaseControl"=w381, "last case"=w379, "event"=w375, "finish?"=TRUE) -> ("CaseControl"=w382:T2, "event"=w380:T1)  [unwired: 14 in]
        n103 = Bundle By Name(cluster=w384, "CaseControl"=w382) -> (w383:T4)
      }
      frame "Write Data Fingereint: 23 F1 F0+26" {
        n104 = Unbundle By Name(w404) -> ("CAN.Write Session in"=w407:refnum<k21>, "CAN.Read Session in"=w406:refnum<k21>, "error"=w405:errorcluster, "CaseControl"=w395:T2)  [unwired: 1 out]
        n105 = Bundle By Name(cluster=T5 {"timestamp"=timestamp(0 s since 1904-01-01), "payload"=[2, 39, 3, 85, 85, 85, 85, 85], "identifier"=402391172, "type"=0, "extended?"=TRUE, "echo?"=FALSE} ("Tx CAN frame"), "payload"=u8[] [3, 241, 240, 38]) -> (w396:T5)
        n106 = call "EOL CAN_Send_Single_Message.vi"("Rx Arbitration Id"=u32 0, "Error in"=w405, "Tx CAN frame"=w396, "Read Session in"=w406, "Write Session in"=w407) -> ("Error out"=w400:errorcluster, "Rx Message"=w401:u8[], "spreadsheet string"=w402:string, "Response Good?"=w391:bool, "TxRx Data"=w398:string[][])  [unwired: 2 in]
        n107 = call "histCase.vi"("CaseControl"=w395, "last case"=w390, "event"=Command."EraseFlashMemory Routine: 31 01 FD 00 44", "finish?"=w391) -> ("CaseControl"=w394:T2, "event"=w393:T1)  [unwired: 14 in]
        n108 = Bundle By Name(cluster=w404, "CAN.TxRx Data"=w398, "CAN.Response Good?"=w391, "CAN.spreadsheet string"=w402, "CAN.Rx Message"=w401, "error"=w400, "CaseControl"=w394) -> (w403:T4)
      }
      frame "EraseFlashMemory Routine: 31 01 FD 00 44" {
        n109 = Unbundle By Name(w423) -> ("CAN.Write Session in"=w426:refnum<k21>, "CAN.Read Session in"=w425:refnum<k21>, "error"=w424:errorcluster, "CaseControl"=w414:T2)  [unwired: 1 out]
        n110 = Bundle By Name(cluster=T5 {"timestamp"=timestamp(0 s since 1904-01-01), "payload"=[2, 39, 3, 85, 85, 85, 85, 85], "identifier"=402391172, "type"=0, "extended?"=TRUE, "echo?"=FALSE} ("Tx CAN frame"), "payload"=u8[] [5, 49, 1, 253, 0, 68]) -> (w415:T5)
        n111 = call "EOL CAN_Send_Single_Message.vi"("Rx Arbitration Id"=u32 0, "Error in"=w424, "Tx CAN frame"=w415, "Read Session in"=w425, "Write Session in"=w426) -> ("Error out"=w419:errorcluster, "Rx Message"=w420:u8[], "spreadsheet string"=w421:string, "Response Good?"=w410:bool, "TxRx Data"=w417:string[][])  [unwired: 2 in]
        n112 = call "histCase.vi"("CaseControl"=w414, "last case"=w409, "event"=Command."More segment?(each file)", "finish?"=w410) -> ("CaseControl"=w413:T2, "event"=w412:T1)  [unwired: 14 in]
        n113 = Bundle By Name(cluster=w423, "CAN.TxRx Data"=w417, "CAN.Response Good?"=w410, "CAN.spreadsheet string"=w421, "CAN.Rx Message"=w420, "error"=w419, "CaseControl"=w413) -> (w422:T4)
      }
      frame "More segment?(each file)" {
        n114 = Unbundle By Name(w437) -> ("CaseControl"=w434:T2, "CAN.Rx Message"=w441:u8[])
        n115 = Index Array(array=w441, index=5 ("索引")) -> (element=w439:u8)
        n116 = Equal?(x=w439, y=0) -> (x = y?=w431:bool)
        n117 = Select(t=Command."Request Download: 34 00 44", s=w431, f=Command."EraseFlashMemory Routine: 31 01 FD 00 44") -> (s? t:f=w428:T1)
        n118 = call "histCase.vi"("CaseControl"=w434, "last case"=w432, "event"=w428, "finish?"=TRUE) -> ("CaseControl"=w435:T2, "event"=w433:T1)  [unwired: 14 in]
        n119 = Bundle By Name(cluster=w437, "CaseControl"=w435) -> (w436:T4)
      }
    }
    n120 = Wait (ms)(milliseconds to wait=u32 10 ("等待时间（毫秒）")) -> ()  [unwired: 1 out]
    n121 = Unbundle By Name(w11) -> ("CaseControl.histCase"=w13:T7)
    n122 = for {
      tunnel: w13 -> [w24] mode=indexing
      shift-right: [w20] -> w12
      shift-left: "" -> [w19]
      n123 = Unbundle By Name(w24) -> ("time"=w22:string, "pass?"=w23:bool, "event"=w18:T1)
      n124 = Format Into String(format string="%S -- %S -- %S\n" ("格式字符串"), initial string=w19, w22, w23, w18) -> (resulting string=w20:string)  [unwired: 1 in, 1 out]
    }
    "Ops" <- w12
  }
